vi "Calculate Forces.vi"(7 "Integrator Reset":bool, 8 "error in (no error)":errorcluster, 10 "Vessel in":refnum<class "Vessel.lvclass">, 11 "Non Linear PID Controller in":refnum<class "Non Linear PID Controller.lvclass">) -> (0 "error out":errorcluster, 2 "Vessel out":refnum<class "Vessel.lvclass">, 3 "Non Linear PID Controller out":refnum<class "Non Linear PID Controller.lvclass">)   [LabVIEW 2014, in "Controller Library.lvlib" / "Non Linear PID Controller.lvclass"]
doc: "This VI calculates the forces in each controlled degree of freedom direction to follow a desired path or point."
uses:
  Non Linear PID Controller.lvclass
  ROV/Vessel.lvclass
  <vilib>/Analysis/Matrix/Datatypes/RealMatrix.ctl
  <vilib>/Analysis/baseanly.llb/A x Vector.vi
  Library/Kinematics/Jinv_euler.vi
  Library/Kinematics/J_euler.vi
  <vilib>/Analysis/Matrix/Numeric/Add/Add - RM,RM.vi
  <vilib>/imath/engines/lvmath2/RunTimeEngine/Managers/WorkSpace/UID Generator.vi
  <vilib>/imath/engines/lvmath2/RunTimeEngine/RunTimeType/NIMS_RunTimeType_From StrictType (excl LVString).vi
  <instcachedir>/0/NIMS_RunTimeType_From StrictType (excl LVString)_15A5391EEA9C4AACB9955AC755B83D29.lvgen/NIMS_RunTimeType_From StrictType (excl LVString)_15A5391EEA9C4AACB9955AC755B83D29_000.vi
  <vilib>/imath/engines/lvmath2/RunTimeEngine/RunTimeType/NIMS_RunTimeType_Set Source Original Bool.vi
  <vilib>/imath/engines/lvmath2/RunTimeEngine/LocalVariableDefStatement/MC_LocalVariableDefStatement_Display.vi
  <vilib>/imath/engines/lvmath2/RunTimeEngine/Managers/SymbolTable/Clear UID.vi
  <vilib>/imath/engines/lvmath2/RunTimeEngine/NodeEndStatement/NIMS_NodeEndStatement_Output.vi
  <instcachedir>/0/NIMS_NodeEndStatement_Output_53EC0D466D134D7ABD903AC30B43404B.lvgen/NIMS_NodeEndStatement_Output_53EC0D466D134D7ABD903AC30B43404B_012.vi
  <vilib>/imath/engines/lvmath2/RunTimeEngine/ErrorHandling/NIMS_Finalize Error.vi
  Library/Integrator/Integrator trapez vector.vi
  <vilib>/Analysis/Matrix/Numeric/Conversions/Matrix To Array - RM.vi
  <vilib>/imath/engines/lvmath2/RunTimeEngine/ArithmeticOperatorToken/NIMS_ArithmeticOperator_multmx(M,CV).vi
  <instcachedir>/0/NIMS_ArithmeticOperator_multmx(M,CV)_787B4652E60B4C52835A7FB23671E425.lvgen/NIMS_ArithmeticOperator_multmx(M,CV)_787B4652E60B4C52835A7FB23671E425_000.vi
  <vilib>/imathl/engines/lvmath/Functions/Error Handling/Create Error.vi
  <vilib>/imath/engines/lvmath2/RunTimeEngine/NodeEndStatement/NIMS_NodeEndStatement_Get Vector.vi
  <instcachedir>/0/NIMS_NodeEndStatement_Get Vector_00D1625602D843AD9D7EC134A9EC13A2.lvgen/NIMS_NodeEndStatement_Get Vector_00D1625602D843AD9D7EC134A9EC13A2_001.vi
  <instcachedir>/0/NIMS_NodeEndStatement_Output_53EC0D466D134D7ABD903AC30B43404B.lvgen/NIMS_NodeEndStatement_Output_53EC0D466D134D7ABD903AC30B43404B_005.vi
  <vilib>/imath/engines/lvmath2/RunTimeEngine/IndexRead/NIMS V(S).vi
  <instcachedir>/0/NIMS V(S)_0488751826AF41519A22953C041130DC.lvgen/NIMS V(S)_0488751826AF41519A22953C041130DC_006.vi
  <vilib>/imath/engines/lvmath2/RunTimeEngine/IndexReplace/NIMS V(S)=S.vi
  <instcachedir>/0/NIMS V(S)=S_2D52C4EC15D8415E870AEE69FB516CCA.lvgen/NIMS V(S)=S_2D52C4EC15D8415E870AEE69FB516CCA_000.vi
  <vilib>/imath/engines/lvmath2/RunTimeEngine/BuiltInFunctions/length/NIMS_length(GM).vi
  <instcachedir>/0/NIMS_length(GM)_47CEC356FCE0482D9BA47DC61C99F2C7.lvgen/NIMS_length(GM)_47CEC356FCE0482D9BA47DC61C99F2C7_000.vi
  <vilib>/imath/engines/lvmath2/RunTimeEngine/RangeToken/NIMS_Range_R3 - Integer.vi
  <instcachedir>/0/NIMS_Range_R3 - Integer_66B9031982364693905FDE422E56E490.lvgen/NIMS_Range_R3 - Integer_66B9031982364693905FDE422E56E490_000.vi
  <vilib>/imath/engines/lvmath2/RunTimeEngine/CommandStatement/MC_CommandStatement_break.vi
  <vilib>/imath/engines/lvmath2/RunTimeEngine/IndexRead/NIMS M(S).vi
  <instcachedir>/0/NIMS M(S)_B826C018497E4940AE96BD27B540B6FB.lvgen/NIMS M(S)_B826C018497E4940AE96BD27B540B6FB_000.vi
  <instcachedir>/0/NIMS V(S)_0488751826AF41519A22953C041130DC.lvgen/NIMS V(S)_0488751826AF41519A22953C041130DC_000.vi
  <vilib>/imath/engines/lvmath2/RunTimeEngine/ErrorHandling/NIMS_Create Error From Enums.vi
  <vilib>/imath/engines/lvmath2/RunTimeEngine/IndexReplace/NIMS M(S)=S.vi
  <instcachedir>/0/NIMS M(S)=S_D871EE7B27E5455586ED06C330670F09.lvgen/NIMS M(S)=S_D871EE7B27E5455586ED06C330670F09_001.vi
  <vilib>/imath/engines/lvmath2/RunTimeEngine/ArithmeticOperatorToken/NIMS_ArithmeticOperator_minus.vi
  <instcachedir>/0/NIMS_ArithmeticOperator_minus_39C0593E74DA4138ACA2AB742906488D.lvgen/NIMS_ArithmeticOperator_minus_39C0593E74DA4138ACA2AB742906488D_002.vi
  <vilib>/imath/engines/lvmath/Functions/Error Handling/MergeErrorsWrapper.vi
  Supervisor/Supervisor.lvclass
  <vilib>/Analysis/NI_AALBase.lvlib
  <vilib>/Analysis/Matrix/NI_Matrix.lvlib
  <vilib>/imath/engines/lvmath2/RunTimeEngine/Managers/SymbolTable/NIMS_WorkSpace.lvlib
panel:
  out "Real Matrix":T1
  out "error NU":dbl[](array[numeric])
  out "Heave":cluster{dbl, dbl, dbl, dbl}(graph)
  out "psi_tilde":dbl(graph)
  out "y_tilde":dbl(graph)
  out "x_tilde":dbl(graph)
  out "Yaw":cluster{dbl, dbl, dbl, dbl}(graph)
  out "Sway":cluster{dbl, dbl, dbl, dbl}(graph)
  out "Surge":cluster{dbl, dbl, dbl, dbl}(graph)
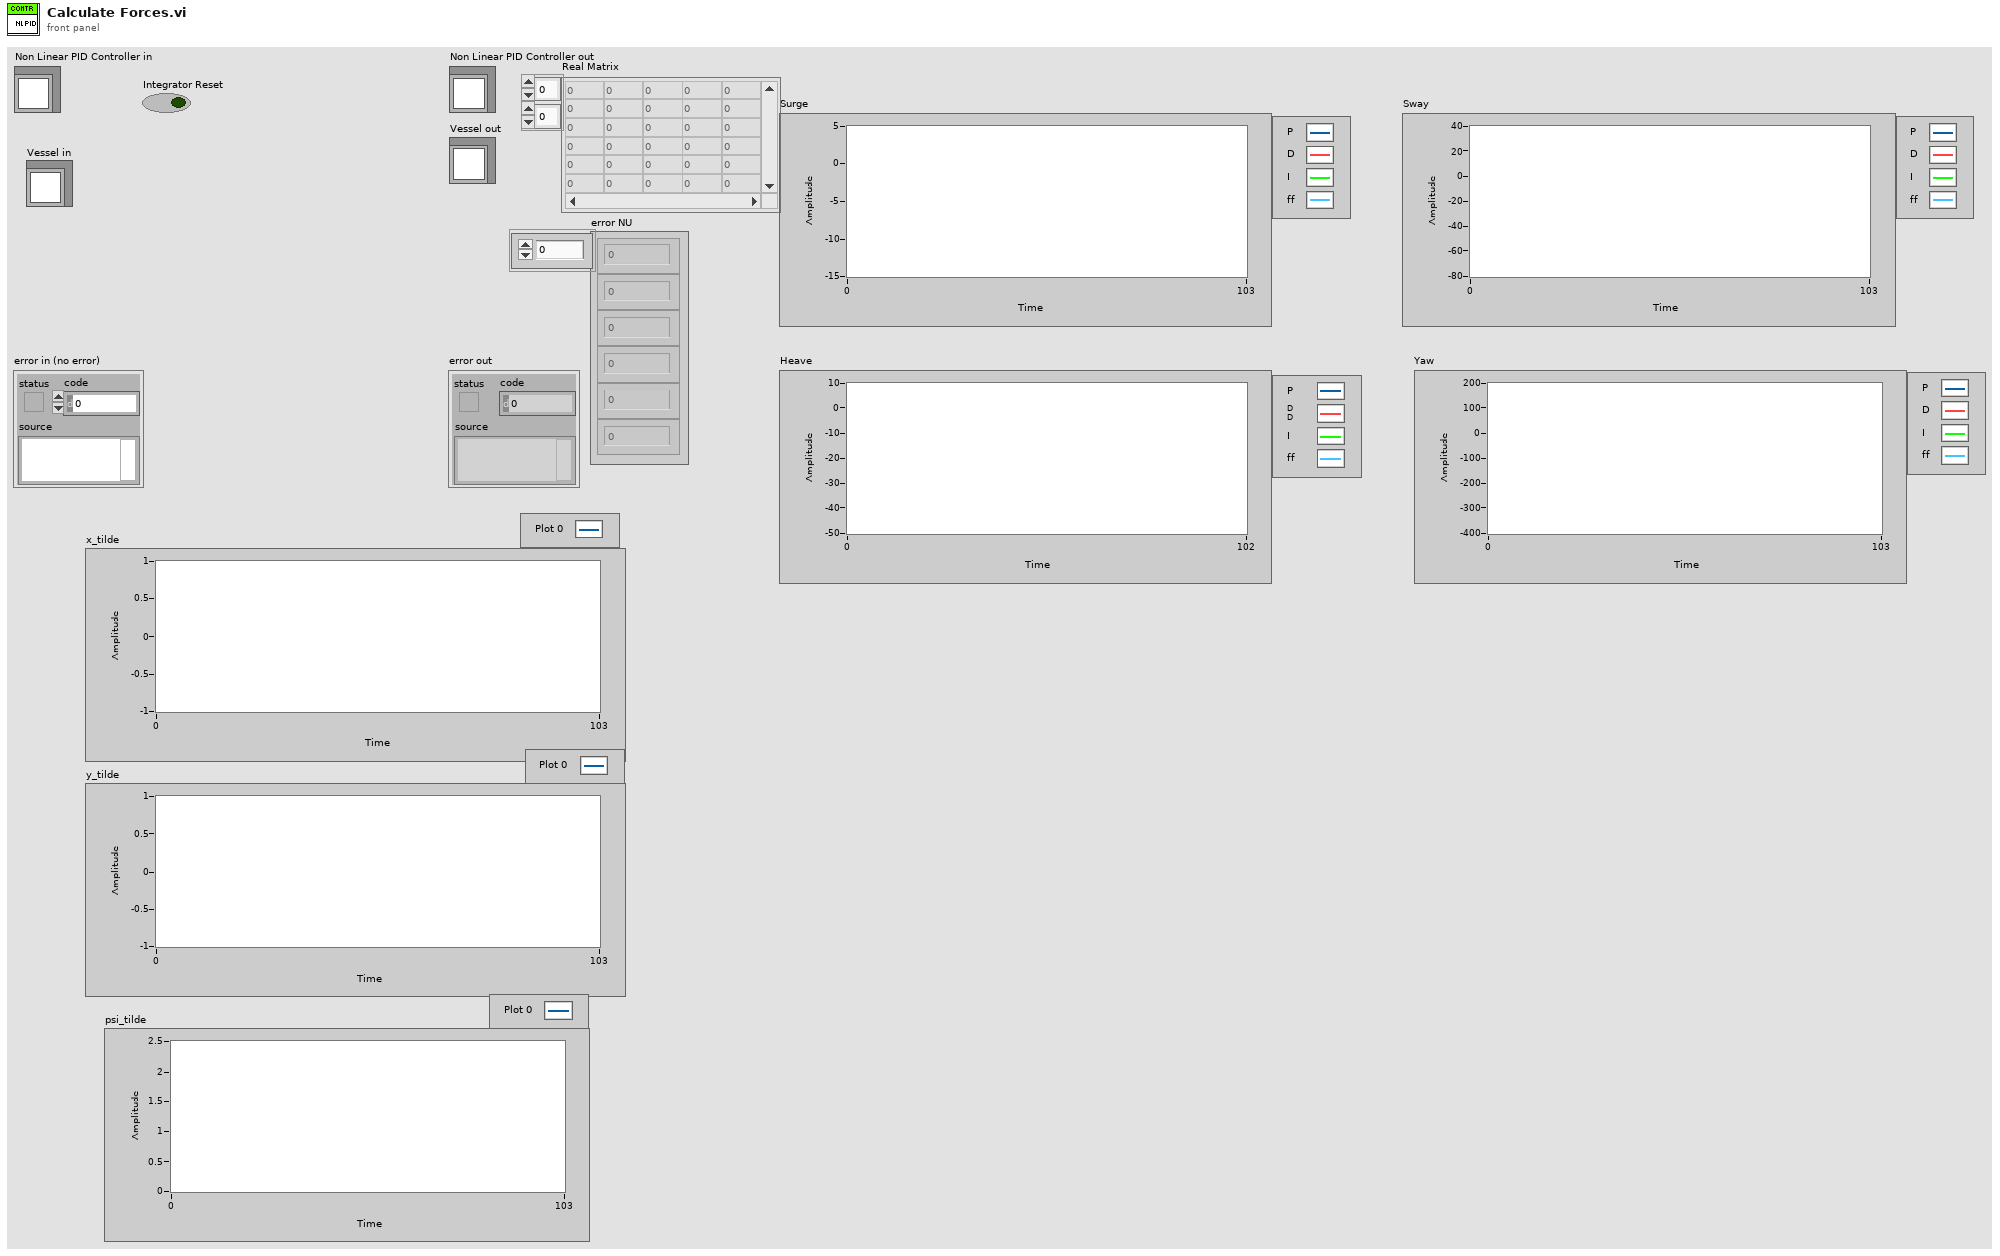
[diagram p1: front panel]
types:
  T1 = typedef "NI_Matrix.lvlib/RealMatrix.ctl" = dbl[][]
  T2 = cluster{"Measured":cluster{"Eta":dbl[], "Nu":dbl[], "Eta Dot":dbl[], "Nu Dot":dbl[]}, "Estimated":cluster{"Eta":dbl[], "Nu":dbl[], "Eta Dot":dbl[], "Nu Dot":dbl[]}, "Desired":cluster{"Eta":dbl[], "Nu":dbl[], "Eta Dot":dbl[], "Nu Dot":dbl[]}, "Previous Desired":cluster{"Eta":dbl[], "Nu":dbl[], "Eta Dot":dbl[], "Nu Dot":dbl[]}, "tau":dbl[], "Altitude":cluster{"Measured":dbl, "Estimated":dbl, "Desired":dbl, "Previous Desired":dbl, "Approximated":dbl, "grad F":dbl[]}, "rpm":dbl[], "Attitude":cluster{"Theta Measured":dbl[], "Theta Estimated":dbl[], "Omega Measured":dbl[], "Omega Estimated":dbl[], "Gyro Bias":dbl[]}}
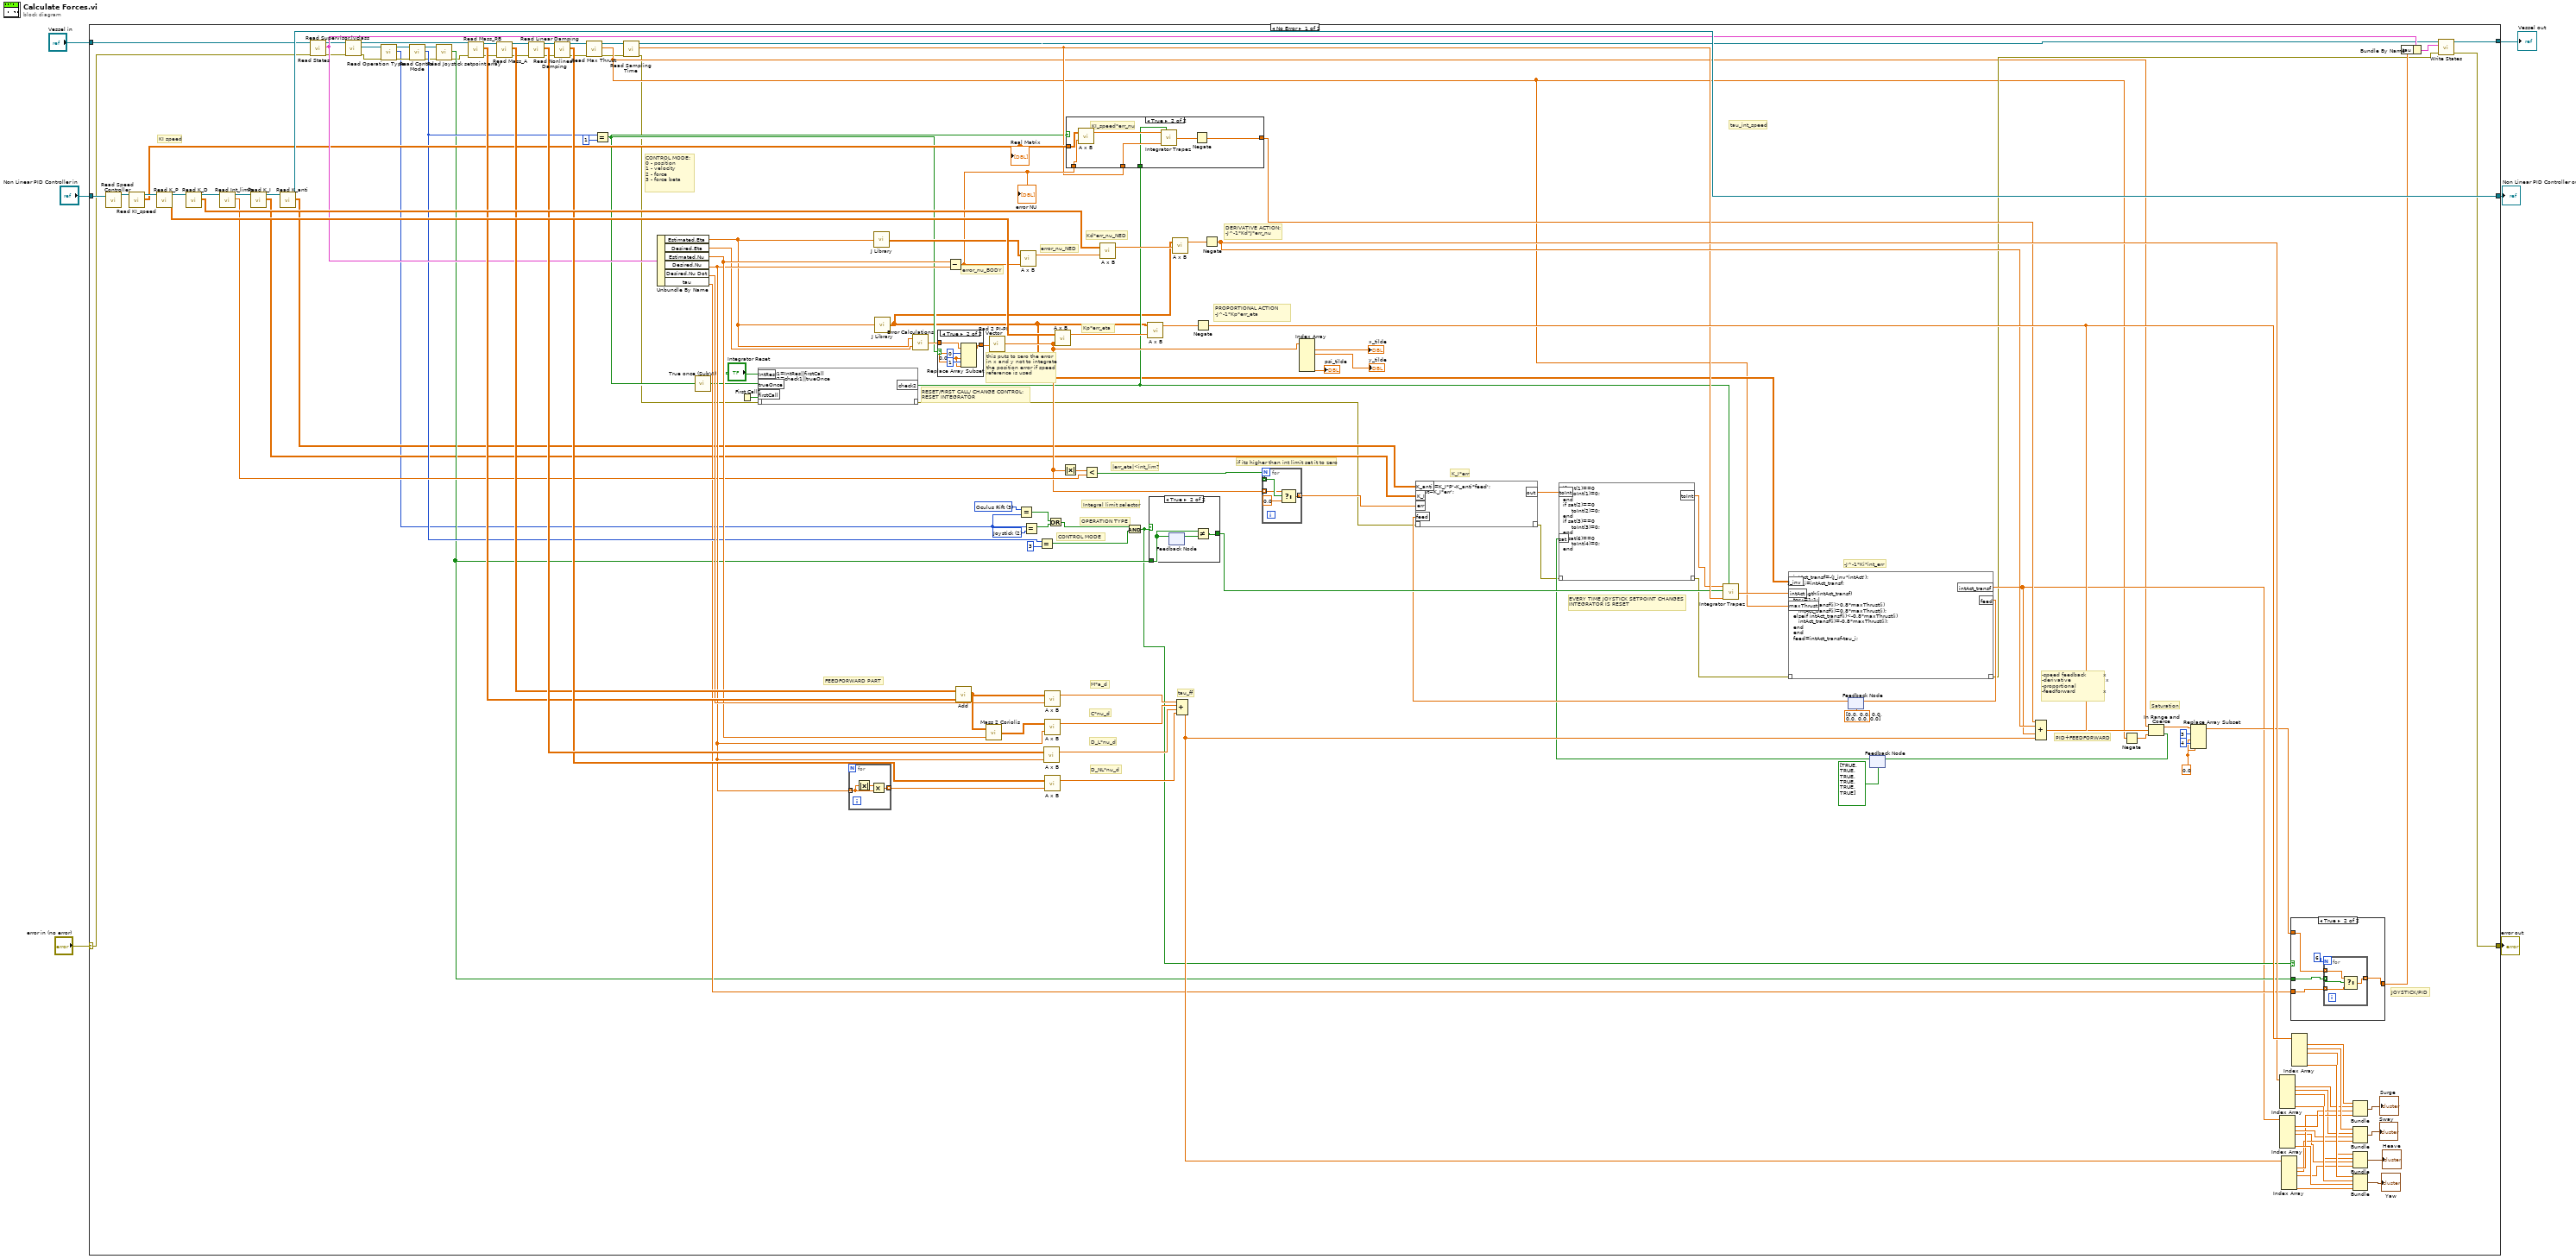
[diagram p0: block diagram]
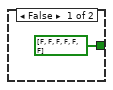
[diagram p2: hidden frame]
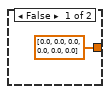
[diagram p5: hidden frame]
diagram:
  n1 = case shown="No Error" "error in (no error)" {
    selector: "error in (no error)" -> [w36 w773]
    tunnel: [w29 w773] -> w5
    tunnel: "Non Linear PID Controller in" -> [w82 w772]
    tunnel: [w120 w772] -> w3
    tunnel: "Vessel in" -> [w119 w771]
    tunnel: [w118 w771] -> w1
    frame No Error {
      w11 = u16 3 items=["Tracking", "DP", "Joystick", "Oculus Rift"] ("Operation Type")
      w51 = u16 2 items=["Tracking", "DP", "Joystick"] ("Operation Type")
      w102 = 0.0 ("new element/subarray")
      # "-speed feedback          x\n-derivative                    x\n-proportional               \n-feedforward                x"
      # "this puts to zero the error in x and y not to integrate the position error if speed reference is used"
      # "KI speed"
      # "EVERY TIME JOYSTICK SETPOINT CHANGES\nINTEGRATOR IS RESET"
      # "PID+FEEDFORWARD"
      # "JOYSTICK/PID"
      # "don't integrate if saturation occurs"
      # "if its higher than int limit set it to zero"
      # "|err_eta|<int_lim?"
      # "CONTROL MODE"
      # "OPERATION TYPE"
      # "RESET/FIRST CALL/ CHANGE CONTROL:\nRESET INTEGRATOR"
      # "PROPORTIONAL ACTION\n-J^-1*Kp*err_eta"
      # "CONTROL MODE:\n0 - position\n1 - velocity\n2 - force\n3 - force beta"
      # "Kp*err_eta"
      # "DERIVATIVE ACTION:\n-J^-1*Kd*J*err_nu"
      # "Kd*err_nu_NED"
      # "error_nu_NED"
      # "error_nu_BODY"
      # "FEEDFORWARD PART"
      # "-J^-1*Ki*int_err"
      # "K_I*err"
      # "tau_int_speed"
      # "Saturation"
      # "tau_ff"
      # "D_NL*nu_d"
      # "D_L*nu_d"
      # "C*nu_d"
      # "M*a_d"
      # "Integral limit selector"
      n2 = call-dynamic "Read Speed Controller.vi"("Non Linear PID Controller in"=w82) -> ("Non Linear PID Controller out"=w81:refnum<class "Non Linear PID Controller.lvclass">)  [unwired: 8 in, 2 out]
      n3 = call-dynamic "Read KI_speed.vi"("Non Linear PID Controller in"=w81) -> ("Real Matrix"=w79:T1, "Non Linear PID Controller out"=w80:refnum<class "Non Linear PID Controller.lvclass">)  [unwired: 8 in, 1 out]
      "Real Matrix" <- w79
      n4 = call-dynamic "Read K_P.vi"("PID Controller in"=w80) -> ("K_P"=w147:T1, "PID Controller out"=w140:refnum<class "Non Linear PID Controller.lvclass">)  [unwired: 8 in, 1 out]
      n5 = call-dynamic "Read K_D.vi"("PID Controller in"=w140) -> ("K_D"=w145:T1, "PID Controller out"=w123:refnum<class "Non Linear PID Controller.lvclass">)  [unwired: 8 in, 1 out]
      n6 = call-dynamic "Read Int_limit.vi"("Non Linear PID Controller in"=w123) -> ("Int_limit"=w109:dbl[], "Non Linear PID Controller out"=w122:refnum<class "Non Linear PID Controller.lvclass">)  [unwired: 8 in, 1 out]
      n7 = call-dynamic "Read K_I.vi"("PID Controller in"=w122) -> ("K_I"=w48:T1, "PID Controller out"=w121:refnum<class "Non Linear PID Controller.lvclass">)  [unwired: 8 in, 1 out]
      n8 = call-dynamic "Read K_anti.vi"("Non Linear PID Controller in"=w121) -> ("K_A"=w47:T1, "Non Linear PID Controller out"=w120:refnum<class "Non Linear PID Controller.lvclass">)  [unwired: 8 in, 1 out]
      n9 = call-dynamic "Read States.vi"("error in (no error)"=w36, "Vessel in"=w119) -> ("error out"=w58:errorcluster, "States"=w114:T2, "Vessel out"=w69:refnum<class "Vessel.lvclass">)  [unwired: 7 in]
      n10 = call "Read Supervisor.lvclass.vi"("error in (no error)"=w58, "Vessel in"=w69) -> ("error out"=w54:errorcluster, "Supervisor.lvclass"=w56:refnum<class "Supervisor.lvclass">, "Vessel out"=w68:refnum<class "Vessel.lvclass">)  [unwired: 7 in]
      n11 = call-dynamic "Read Operation Type.vi"("error in (no error)"=w54, "Supervisor in"=w56) -> ("error out"=w53:errorcluster, "Operation Type"=w10:u16, "Supervisor out"=w55:refnum<class "Supervisor.lvclass">)  [unwired: 7 in]
      n12 = call-dynamic "Read Control Mode.vi"("error in (no error)"=w53, "Supervisor in"=w55) -> ("error out"=w59:errorcluster, "Control Mode"=w64:u16, "Supervisor out"=w60:refnum<class "Supervisor.lvclass">)  [unwired: 7 in]
      n13 = call-dynamic "Read Joystick setpoint array.vi"("error in (no error)"=w59, "Supervisor in"=w60) -> ("error out"=w35:errorcluster, "Joystick setpoint array"=w57:bool[])  [unwired: 7 in, 1 out]
      n14 = call "Read Mass_RB.vi"("error in (no error)"=w35, "Vessel in"=w68) -> ("error out"=w34:errorcluster, "Mass"=w125:T1, "Vessel out"=w128:refnum<class "Vessel.lvclass">)  [unwired: 7 in]
      n15 = call "Read Mass_A.vi"("error in (no error)"=w34, "Vessel in"=w128) -> ("error out"=w33:errorcluster, "Added Mass"=w126:T1, "Vessel out"=w127:refnum<class "Vessel.lvclass">)  [unwired: 7 in]
      n16 = call "Read Linear Damping.vi"("error in (no error)"=w33, "Vessel in"=w127) -> ("error out"=w32:errorcluster, "Real Matrix"=w135:T1, "Vessel out"=w148:refnum<class "Vessel.lvclass">)  [unwired: 7 in]
      n17 = call "Read Nonlinear Damping.vi"("error in (no error)"=w32, "Vessel in"=w148) -> ("error out"=w20:errorcluster, "Real Matrix"=w133:T1, "Vessel out"=w138:refnum<class "Vessel.lvclass">)  [unwired: 7 in]
      n18 = call "Read Max Thrust.vi"("error in (no error)"=w20, "Vessel in"=w138) -> ("error out"=w19:errorcluster, "Max Thrust"=w21:dbl[], "Vessel out"=w112:refnum<class "Vessel.lvclass">)  [unwired: 7 in]
      n19 = Equal?(x=w64, y=u16 1) -> (x = y?=w66:bool)
      n20 = call-dynamic "Read Sampling Time.vi"("error in (no error)"=w19, "Vessel in"=w112) -> ("error out"=w18:errorcluster, "Sampling Time"=w77:dbl, "Vessel out"=w111:refnum<class "Vessel.lvclass">)  [unwired: 7 in]
      n21 = Unbundle By Name(w114) -> ("Estimated.Eta"=w108:dbl[], "Desired.Eta"=w107:dbl[], "Estimated.Nu"=w116:dbl[], "Desired.Nu"=w115:dbl[], "Desired.Nu Dot"=w117:dbl[], "tau"=w63:dbl[])
      n22 = call "True once (SubVI).vi"("Automatic"=w66) -> ("Boolean"=w44:bool)
      n23 = First Call?() -> (First Call?: T/F=w42:bool)
      n24 = mathscript code="check1=IntRes||firstCall\ncheck2=check1||trueOnce"("??"=w18, "IntRes"="Integrator Reset", "trueOnce"=w44, "firstCall"=w42) -> ("??"=w31:errorcluster, "check2"=w41:bool)
      n25 = for {
        tunnel: w115 -> [w765] mode=indexing
        tunnel: [w766] -> w134 mode=indexing
        n26 = Absolute Value(x=w765) -> (abs(x)=w764:dbl)
        n27 = Multiply(x=w764, y=w765) -> (x*y=w766:dbl)
      }
      n28 = call-poly "J Library.vi"("eta"=w108) -> ("J"=w110:T1)
      n29 = call-poly "J Library.vi"("eta"=w108) -> ("Jinv"=w40:T1)
      n30 = call "Error Calculations.vi"("Eta_ref"=w107, "Eta"=w108) -> ("error"=w71:dbl[])
      n31 = case shown="True" w66 {
        tunnel: w71 -> [w750 w755]
        tunnel: [w750 w754] -> w70
        frame False {
        }
        frame True {
          w751 = 0.0 ("new element/subarray")
          n32 = Replace Array Subset(array=w755, new element #1=w751, index #1=0 ("index"), new element #2=w751, index #2=1 ("index")) -> (w754:dbl[])
        }
      }
      n33 = Subtract(x=w116, y=w115) -> (x-y=w78:dbl[])
      "error NU" <- w78
      n34 = call-poly <vilib>:"Add.vi"("Real Matrix B"=w125, "Real Matrix A"=w126) -> ("A + B"=w124:T1)
      n35 = call "Mass 2 Coriolis.vi"("nu"=w116, "M"=w124) -> ("C"=w136:T1)
      n36 = call "Rad 2 PI-PI Vector.vi"("vector in"=w70) -> ("vector out"=w86:dbl[])
      n37 = Equal?(x=w11, y=w10) -> (x = y?=w9:bool)
      n38 = call-poly <vilib>:"A x B.vi"("Vector"=w78, "A"=w110) -> ("A x Vector"=w146:dbl[])  [unwired: 1 out]
      n39 = Equal?(x=w10, y=w51) -> (x = y?=w8:bool)
      n40 = Equal?(x=w64, y=u16 3) -> (x = y?=w52:bool)
      n41 = call-poly <vilib>:"A x B.vi"("Vector"=w115, "A"=w135) -> ("A x Vector"=w131:dbl[])  [unwired: 1 out]
      n42 = call-poly <vilib>:"A x B.vi"("Vector"=w117, "A"=w124) -> ("A x Vector"=w129:dbl[])  [unwired: 1 out]
      n43 = call-poly <vilib>:"A x B.vi"("Vector"=w115, "A"=w136) -> ("A x Vector"=w130:dbl[])  [unwired: 1 out]
      n44 = call-poly <vilib>:"A x B.vi"("Vector"=w134, "A"=w133) -> ("A x Vector"=w132:dbl[])  [unwired: 1 out]
      n45 = Or(x=w9, y=w8) -> (x .or. y?=w7:bool)
      n46 = call-poly <vilib>:"A x B.vi"("Vector"=w86, "A"=w147) -> ("A x Vector"=w106:dbl[])  [unwired: 1 out]
      n47 = Absolute Value(x=w86) -> (abs(x)=w141:dbl[])
      n48 = case shown="True" w66 {
        tunnel: w79 -> [_ w763]
        tunnel: w78 -> [_ w762]
        tunnel: w77 -> [_ w760]
        tunnel: w41 -> [_ w759]
        tunnel: [dbl[] [0.0, 0.0, 0.0, 0.0, 0.0, 0.0] w757] -> w76
        frame False {
        }
        frame True {
          # "KI_speed*err_nu"
          n49 = call-poly <vilib>:"A x B.vi"("Vector"=w762, "A"=w763) -> ("A x Vector"=w761:dbl[])  [unwired: 1 out]
          n50 = call-poly "Integrator Trapez.vi"("Reset"=w759, "dt"=w760, "Input"=w761) -> ("Output"=w758:dbl[])  [unwired: 3 in]
          n51 = Negate(x=w758) -> (-x=w757:dbl[])
        }
      }
      n52 = Less?(x=w141, y=w109) -> (x < y?=w139:bool[])
      n53 = call-poly <vilib>:"A x B.vi"("Vector"=w146, "A"=w145) -> ("A x Vector"=w144:dbl[])  [unwired: 1 out]
      n54 = And(x=w7, y=w52) -> (x .and. y?=w50:bool)
      n55 = call-poly <vilib>:"A x B.vi"("Vector"=w106, "A"=w40) -> ("A x Vector"=w142:dbl[])  [unwired: 1 out]
      n56 = case shown="True" w50 {
        tunnel: w57 -> [_ w738]
        tunnel: [bool[] [FALSE, FALSE, FALSE, FALSE, FALSE, FALSE] w737] -> w49
        frame False {
        }
        frame True {
          n57 = feedback #1() -> (w739:bool[])  [unwired: 1 in]
          n58 = feedback-in #1(w738) -> ()
          n59 = Not Equal?(x=w738, y=w739) -> (x != y?=w737:bool[])
        }
      }
      n60 = call-poly <vilib>:"A x B.vi"("Vector"=w144, "A"=w40) -> ("A x Vector"=w143:dbl[])  [unwired: 1 out]
      n61 = Compound Arithmetic op=ADD(w129, w130, w131, w132) -> (w92:dbl[])
      n62 = Negate(x=w142) -> (-x=w101:dbl[])
      n63 = Negate(x=w143) -> (-x=w97:dbl[])
      n64 = for {
        tunnel: w139 -> [w770] mode=indexing
        tunnel: w86 -> [w769] mode=indexing
        tunnel: [w767] -> w45 mode=indexing
        n65 = Select(t=w769, s=w770, f=0.0) -> (s? t:f=w767:dbl)
      }
      n66 = Index Array(array=w86) -> (element #1=→"x_tilde":dbl, element #2=→"y_tilde":dbl, element #6=→"psi_tilde":dbl)  [unwired: 6 in, 3 out]
      n67 = feedback #2(dbl[] [0.0, 0.0, 0.0, 0.0, 0.0, 0.0]) -> (w46:dbl[])
      n68 = mathscript code="%out=K_I*P'-K_anti*feed';\nout=K_I*err';"("??"=w31, "K_I"=w48, "err"=w45, "K_anti"=w47, "feed"=w46) -> ("??"=w24:errorcluster, "out"=w27:dbl[])
      n69 = feedback #3(bool[] [TRUE, TRUE, TRUE, TRUE, TRUE, TRUE]) -> (w26:bool[])
      n70 = mathscript code="if sat(1)==0\n     toInt(1)=0;\nend\nif sat(2)==0\n     toInt(2)=0;\nend\nif sat(3)==0\n     toInt(3)=0;\nend\nif sat(6)==0\n     toInt(4)=0;\nend"("??"=w24, "toInt"=w27, "sat"=w26) -> ("??"=w23:errorcluster, "toInt"=w28:dbl[])
      n71 = call-poly "Integrator Trapez.vi"("Reset"=w41, "dt"=w77, "Reset Array"=w49, "Input"=w28) -> ("Output"=w39:dbl[])  [unwired: 2 in]
      n72 = mathscript code="intAct_transf=-(J_inv*intAct');\ntau_i=intAct_transf;\n\nl=length(intAct_transf)\nfor i=1:1:l\nif intAct_transf(i)>0.8*maxThrust(i)\n   intAct_transf(i)=0.8*maxThrust(i);\nelseif intAct_transf(i)<-0.8*maxThrust(i)\n   intAct_transf(i)=-0.8*maxThrust(i);\nend\nend\nfeed=intAct_transf-tau_i;"("??"=w23, "J_inv"=w40, "intAct"=w39, "maxThrust"=w21) -> ("??"=w30:errorcluster, "intAct_transf"=w38:dbl[], "feed"=w37:dbl[])
      n73 = feedback-in #2(w37) -> ()
      n74 = Compound Arithmetic op=ADD(w76, w97, w101, w38, w92) -> (w22:dbl[])
      n75 = Negate(x=w21) -> (-x=w12:dbl[])
      n76 = In Range and Coerce(upper limit=w21, x=w22, lower limit=w12) -> (coerced(x)=w105:dbl[], In Range?=w13:bool[])
      n77 = feedback-in #3(w13) -> ()
      n78 = Replace Array Subset(array=w105, new element #1=w102, index #1=3 ("index"), new element #2=w102, index #2=4 ("index")) -> (w62:dbl[])
      n79 = Index Array(array=w97) -> (element #1=w17:dbl, element #2=w16:dbl, element #3=w74:dbl, element #6=w96:dbl)  [unwired: 6 in, 2 out]
      n80 = Index Array(array=w38) -> (element #1=w95:dbl, element #2=w94:dbl, element #3=w15:dbl, element #6=w93:dbl)  [unwired: 6 in, 2 out]
      n81 = Index Array(array=w92) -> (element #1=w91:dbl, element #2=w90:dbl, element #3=w73:dbl, element #6=w14:dbl)  [unwired: 6 in, 2 out]
      n82 = case shown="True" w50 {
        tunnel: w63 -> [_ w742]
        tunnel: w62 -> [w740 w743]
        tunnel: [w740 w741] -> w61
        tunnel: w57 -> [_ w744]
        frame False {
        }
        frame True {
          n83 = for {
            N: 6 -> [_]
            tunnel: [w749] -> w741 mode=indexing
            tunnel: w744 -> [w748] mode=indexing
            tunnel: w743 -> [w747] mode=indexing
            tunnel: w742 -> [w746] mode=indexing
            n84 = Select(t=w747, s=w748, f=w746) -> (s? t:f=w749:dbl)
          }
        }
      }
      n85 = Index Array(array=w101) -> (element #1=w100:dbl, element #2=w99:dbl, element #3=w75:dbl, element #6=w98:dbl)  [unwired: 6 in, 2 out]
      n86 = Bundle(w100, w17, w95, w91) -> (→"Surge":cluster{dbl, dbl, dbl, dbl})  [unwired: 1 in]
      n87 = Bundle(w99, w16, w94, w90) -> (→"Sway":cluster{dbl, dbl, dbl, dbl})  [unwired: 1 in]
      n88 = Bundle(w75, w74, w15, w73) -> (→"Heave":cluster{dbl, dbl, dbl, dbl})  [unwired: 1 in]
      n89 = Bundle(w98, w96, w93, w14) -> (→"Yaw":cluster{dbl, dbl, dbl, dbl})  [unwired: 1 in]
      n90 = Bundle By Name(cluster=w114, "tau"=w61) -> (w113:T2)
      n91 = call-dynamic "Write States.vi"("error in (no error)"=w30, "States"=w113, "Vessel in"=w111) -> ("error out"=w29:errorcluster, "Vessel out"=w118:refnum<class "Vessel.lvclass">)  [unwired: 7 in]
    }
    frame Error {
    }
  }
  "error out" <- w5
  "Non Linear PID Controller out" <- w3
  "Vessel out" <- w1
